vi "Read Cores.vi"(8 "error in (no error)":errorcluster, 11 "ConfigProc in":refnum<class "ConfigProc.lvclass">) -> (0 "error out":errorcluster, 2 "Cores":dbl, 3 "ConfigProc out":refnum<class "ConfigProc.lvclass">)   [LabVIEW 2017, in "ConfigProc.lvclass"]
uses:
  ConfigProc.lvclass
  ConfigProc.lvclass/ConfigProc.ctl
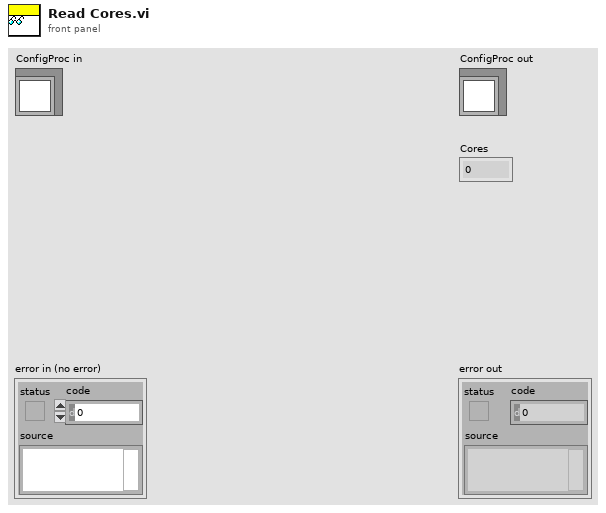
[diagram p1: front panel]
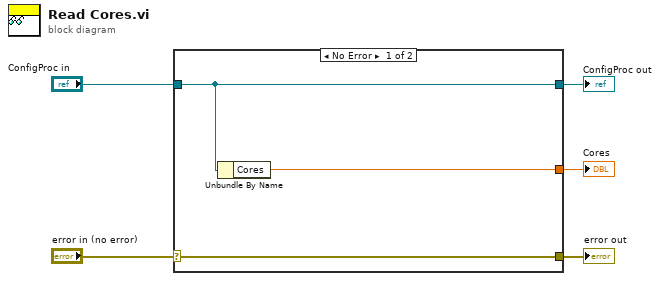
[diagram p0: block diagram]
diagram:
  n1 = case shown="No Error" "error in (no error)" {
    selector: "error in (no error)" -> [w8 w9]
    tunnel: [w8 w9] -> w4
    tunnel: [w7 w10] -> w2
    tunnel: "ConfigProc in" -> [w7 w10]
    tunnel: [w6 _] -> w1
    frame No Error {
      n2 = Unbundle By Name(w7) -> ("Cores"=w6:dbl)
    }
    frame Error {
    }
  }
  "error out" <- w4
  "ConfigProc out" <- w2
  "Cores" <- w1
